vi "TestAll.vi"() -> ()   [LabVIEW 2016]
uses:
  Displacement/DisplacementErrorCodes.ctl
  Inclinometer/InclinometerErrorCodes.ctl
  Telemetry/TelemetryFields.ctl
  <vilib>/rvi/Emulation/niFpgaGetClockAttributes.vi
  <vilib>/rvi/Emulation/niFpgaSctlEmulationGetInTimedLoop.vi
  <vilib>/rvi/Emulation/niFpgaEmulationReportErrorSimple.vi
  <vilib>/rvi/Emulation/niFpgaProcessEmulError.vi
  <vilib>/rvi/Emulation/niFpgaEmulationIsFPGAContextNoSignature.vi
  <vilib>/rvi/errors/niFpgaSetErrorForExecOnDevCompSimple.vi
  <vilib>/rvi/eio/common/nirviEmuReportErrorAndStop.vi
  <vilib>/rvi/DataTransferAndStorage/Container/Common/niFpgaContainerGetUniqueNameForEmu.vi
  <vilib>/rvi/FIFO/Fifo_Resource/nirvififoEmulationSetSize.vi
  <vilib>/rvi/FIFO/Fifo_Resource/nirviFifoEmulationQueueMgr.vi
  <instcachedir>/0/nirviFifoEmulationQueueMgr_E5CAEC123FF24DC58D834DCA3CDAA9B5.lvgen/nirviFifoEmulationQueueMgr_E5CAEC123FF24DC58D834DCA3CDAA9B5_004.vi
  <vilib>/rvi/FIFO/Fifo_Resource/nirvififoEmulationDetermineInputValidOut.vi
  <vilib>/rvi/FIFO/Fifo_Resource/nirvififoEmulationCreateLock.vi
  <vilib>/rvi/FIFO/Fifo_Resource/nirvififoEmulationObtainLock.vi
  <vilib>/rvi/FIFO/Fifo_Resource/nirvififoEmulationReleaseLock.vi
  <vilib>/rvi/occurrence/nirviWaitOnOccurrenceBase.vi
  <vilib>/rvi/errors/nirviReportUnexpectedCaseInternalError.vi
  <vilib>/rvi/errors/nirviReportUnexpectedCaseInternalError (U32).vi
  <vilib>/Utility/error.llb/Clear Errors.vi
  <vilib>/rvi/Emulation/niFpgaCriticalErrorInLSC.vi
  <vilib>/rvi/Memory/Memory_Emulation/nirvimemoryFastEmulation.vi
  <vilib>/rvi/Memory/Memory_Emulation/nirvimemoryEmulation.vi
  <vilib>/rvi/DataTransferAndStorage/Container/Common/niFpgaContainerExecOnDevCompGetState.vi
  <vilib>/rvi/Memory/Memory_Emulation/niFpgaMemoryEmulationCacheClearOnFirstRun.vi
  <vilib>/rvi/Memory/Memory_Emulation/nirvimemoryEmulationManagerCache_MakeExclusive.vi
  <vilib>/rvi/Memory/Memory_Emulation/niFpgaMemoryEmulationValidateCache.vi
  <vilib>/rvi/Memory/Memory_Emulation/nirvimemoryEmulationManagerCache_InsertValue.vi
  <vilib>/rvi/Memory/Memory_Emulation/nirvimemoryEmulationManagerCache_ReleaseExclusive.vi
  <vilib>/rvi/Memory/Memory_Emulation/nirvimemoryEmulationManagerCache_GetValue.vi
  <vilib>/rvi/Memory/Memory_Emulation/nirvimemoryEmulationManagerCache_SetValue.vi
  <vilib>/rvi/Emulation/niFpgaSctlEmulationResourceMgr.vi
  <instcachedir>/0/nirviFifoEmulationQueueMgr_E5CAEC123FF24DC58D834DCA3CDAA9B5.lvgen/nirviFifoEmulationQueueMgr_E5CAEC123FF24DC58D834DCA3CDAA9B5_043.vi
  <instcachedir>/0/nirviFifoEmulationQueueMgr_E5CAEC123FF24DC58D834DCA3CDAA9B5.lvgen/nirviFifoEmulationQueueMgr_E5CAEC123FF24DC58D834DCA3CDAA9B5_040.vi
  <instcachedir>/0/nirviFifoEmulationQueueMgr_E5CAEC123FF24DC58D834DCA3CDAA9B5.lvgen/nirviFifoEmulationQueueMgr_E5CAEC123FF24DC58D834DCA3CDAA9B5_041.vi
  <instcachedir>/0/nirviFifoEmulationQueueMgr_E5CAEC123FF24DC58D834DCA3CDAA9B5.lvgen/nirviFifoEmulationQueueMgr_E5CAEC123FF24DC58D834DCA3CDAA9B5_042.vi
  <instcachedir>/0/nirviFifoEmulationQueueMgr_E5CAEC123FF24DC58D834DCA3CDAA9B5.lvgen/nirviFifoEmulationQueueMgr_E5CAEC123FF24DC58D834DCA3CDAA9B5_038.vi
  <vilib>/rvi/DataTransferAndStorage/Container/XNode/niFpgaContainer.xnode
  <vilib>/rvi/FIFO/Fifo_Resource/nirvififoEmulationWrite.vi
  <vilib>/rvi/FIFO/Fifo_Resource/nirvififoEmulationRead.vi
  <vilib>/rvi/Memory/Memory_Emulation/niFpgaMemoryEmulationRefIn.vi
panel:
  out "Step":i32
  out "Iteration":i32
  out "InclinometerErrorCodeTimestamp":u64
  out "InclinometerSampleTimestamp":u64
  out "InclinometerRxFrames":u64
  out "InclinometerTxFrames":u64
  out "InclinometerRxBytes":u64
  out "InclinometerTxBytes":u64
  out "InclinometerZenithAngle":sgl
  out "InclinometerRawAngle":u32
  out "InclinometerErrorCode":T1
  out "DisplacementErrorCode":T2
  out "DisplacementErrorTimestamp":u64
  out "DisplacementRotationZ":sgl
  out "DisplacementRotationY":sgl
  out "DisplacementRotationX":sgl
  out "DisplacementPositionZ":sgl
  out "DisplacementPositionY":sgl
  out "DisplacementPositionX":sgl
  out "DisplacementEng8":sgl
  out "DisplacementEng7":sgl
  out "DisplacementEng6":sgl
  out "DisplacementEng5":sgl
  out "DisplacementEng4":sgl
  out "DisplacementEng3":sgl
  out "DisplacementEng2":sgl
  out "DisplacementEng1":sgl
  out "DisplacementRaw8":i32
  out "DisplacementRaw7":i32
  out "DisplacementRaw6":i32
  out "DisplacementRaw5":i32
  out "DisplacementRaw4":i32
  out "DisplacementRaw3":i32
  out "DisplacementRaw2":i32
  out "DisplacementRaw1":i32
  out "DisplacementSampleTimestamp":u64
  out "DisplacementRxFrames":u64
  out "DisplacementTxFrames":u64
  out "DisplacementRxBytes":u64
  out "DisplacementTxBytes":u64
  out "AngularAccelerationZ":sgl format="%#.6f"
  out "AngularAccelerationY":sgl format="%#.6f"
  out "AngularAccelerationX":sgl format="%#.6f"
  out "AccelerometerEng8":sgl format="%#.6f"
  out "AccelerometerEng7":sgl format="%#.6f"
  out "AccelerometerEng6":sgl format="%#.6f"
  out "AccelerometerEng5":sgl format="%#.6f"
  out "AccelerometerEng4":sgl format="%#.6f"
  out "AccelerometerEng3":sgl format="%#.6f"
  out "AccelerometerEng2":sgl format="%#.6f"
  out "AccelerometerEng1":sgl format="%#.6f"
  out "AccelerometerTimestamp":u64
  out "AccelerometerRaw1":sgl format="%#.6f"
  out "AccelerometerRaw2":sgl format="%#.6f"
  out "AccelerometerRaw3":sgl format="%#.6f"
  out "AccelerometerRaw4":sgl format="%#.6f"
  out "AccelerometerRaw5":sgl format="%#.6f"
  out "AccelerometerRaw6":sgl format="%#.6f"
  out "AccelerometerRaw7":sgl format="%#.6f"
  out "AccelerometerRaw8":sgl format="%#.6f"
  out "AccelerometerSampleCount":u64
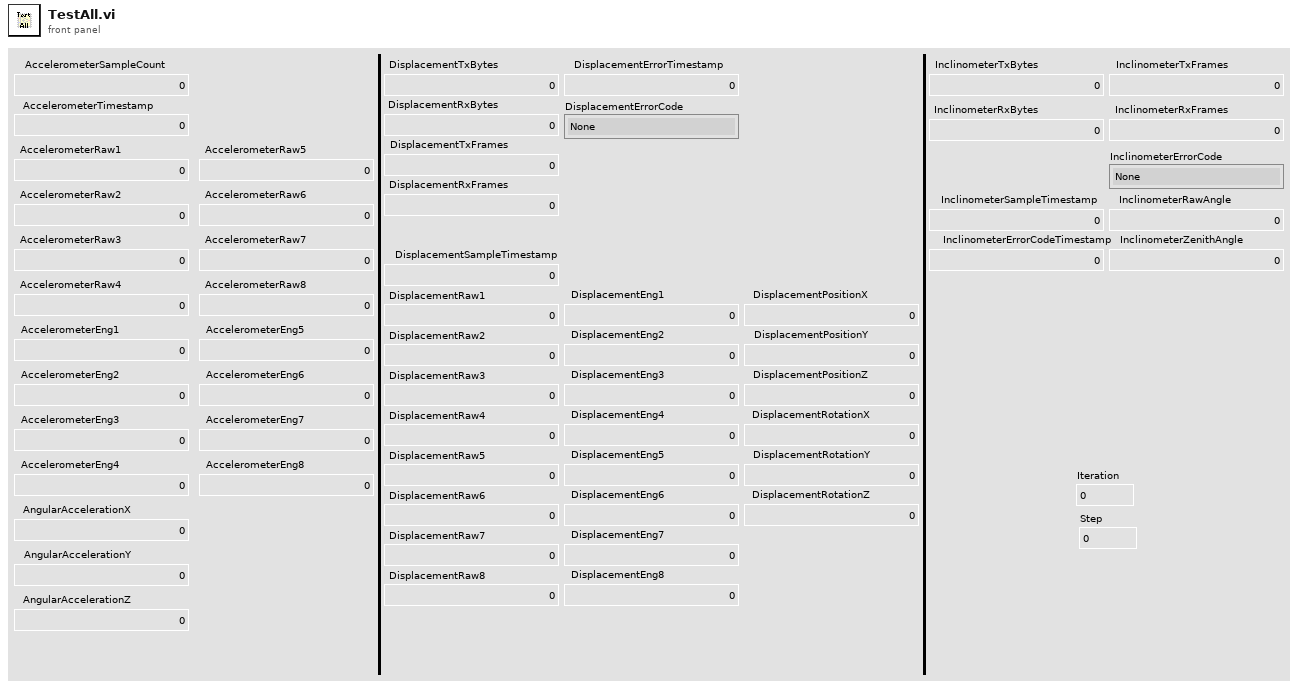
[diagram p1: front panel]
types:
  T1 = typedef "InclinometerErrorCodes.ctl" = enum8{"None", "ResponseAddressError", "ResponseFunctionCodeError", "ResponseByteCountError", "ResponseCRCError", "ResponseUnknownError", "ResponseTimeoutError", "SensorReportsIllegalFunction", "SensorReportsIllegalDataAddress"}
  T2 = typedef "DisplacementErrorCodes.ctl" = enum16{"None", "ResponseUnknownError", "ResponseInvalidError", "ResponseTimeoutError", "SensorIndicatesInvalidCommandError", "SensorIndicatesCommunicationTimeoutError", "SensorIndicatesDataLengthError", "SensorIndicatesNumberOfParametersError", "SensorIndicatesParameterError", "SensorIndicatesCommunicationError", "SensorIndicatesIDNumberError", "SensorIndicatesExpansionLineError", "SensorIndicatesWriteControlError"}
  T3 = cluster{"Timestamp":u64, "TxBytes":u64, "RxBytes":u64, "TxFrames":u64, "RxFrames":u64, "GyroX":u32, "GyroY":u32, "GyroZ":u32, "Status":u8, "SequenceNumber":u8, "Temperature":i16}
  T4 = cluster{"Timestamp":u64, "TxBytes":u64, "RxBytes":u64, "TxFrames":u64, "RxFrames":u64, "BIT0":u8, "BIT1":u8, "BIT2":u8, "BIT3":u8, "BIT4":u8, "BIT5":u8, "BIT6":u8, "BIT7":u8}
  T5 = cluster{"Timestamp":u64, "TxBytes":u64, "RxBytes":u64, "TxFrames":u64, "RxFrames":u64, "BIT0":u8, "BIT1":u8, "BIT2":u8, "BIT3":u8, "BIT4":u8, "BIT5":u8}
  T6 = cluster{"Timestamp":u64, "TxBytes":u64, "RxBytes":u64, "TxFrames":u64, "RxFrames":u64, "ErrorCode":enum8{"None", "ResponseHeaderError", "ResponseCRCError", "ResponseTimeoutError", "ResponseChecksumError"}}
  T7 = typedef "TelemetryFields.ctl" = enum16{"None", "InclinometerTxBytes", "InclinometerRxBytes", "InclinometerTxFrames", "InclinometerRxFrames", "InclinometerErrorTimestamp", "InclinometerErrorCode", "InclinometerSampleTimestamp", "InclinometerRawAngle", "InclinometerZenithAngle", "DisplacementTxBytes", "DisplacementRxBytes", "DisplacementTxFrames", "DisplacementRxFrames", "DisplacementErrorTimestamp", "DisplacementErrorCode", "DisplacementSampleTimestamp", "DisplacementRaw1", "DisplacementRaw2", "DisplacementRaw3", "DisplacementRaw4", "DisplacementRaw5", "DisplacementRaw6", "DisplacementRaw7", "DisplacementRaw8", "DisplacementEng1", "DisplacementEng2", "DisplacementEng3", "DisplacementEng4", "DisplacementEng5", "DisplacementEng6", "DisplacementEng7", "DisplacementEng8", "DisplacementPositionX", "DisplacementPositionY", "DisplacementPositionZ", "DisplacementRotationX", "DisplacementRotationY", "DisplacementRotationZ", "AccelerometerSampleCount", "AccelerometerSampleTimestamp", "AccelerometerRaw1", "AccelerometerRaw2", "AccelerometerRaw3", "AccelerometerRaw4", "AccelerometerRaw5", "AccelerometerRaw6", "AccelerometerRaw7", "AccelerometerRaw8", "AccelerometerEng1", "AccelerometerEng2", "AccelerometerEng3", "AccelerometerEng4", "AccelerometerEng5", "AccelerometerEng6", "AccelerometerEng7", "AccelerometerEng8", "AngularAccelerationX", "AngularAccelerationY", "AngularAccelerationZ", "GyroTxBytes", "GyroRxBytes", "GyroTxFrames", "GyroRxFrames", "GyroErrorTimestamp", "GyroErrorCode", "GyroSampleTimestamp", "AngularVelocityX", "AngularVelocityY", "AngularVelocityZ", "GyroStatus", "GyroSequenceNumber", "GyroTemperature", "GyroBITTimestamp", "GyroBIT0", "GyroBIT1", "GyroBIT2", "GyroBIT3", "GyroBIT4", "GyroBIT5", "GyroBIT6", "GyroBIT7"}
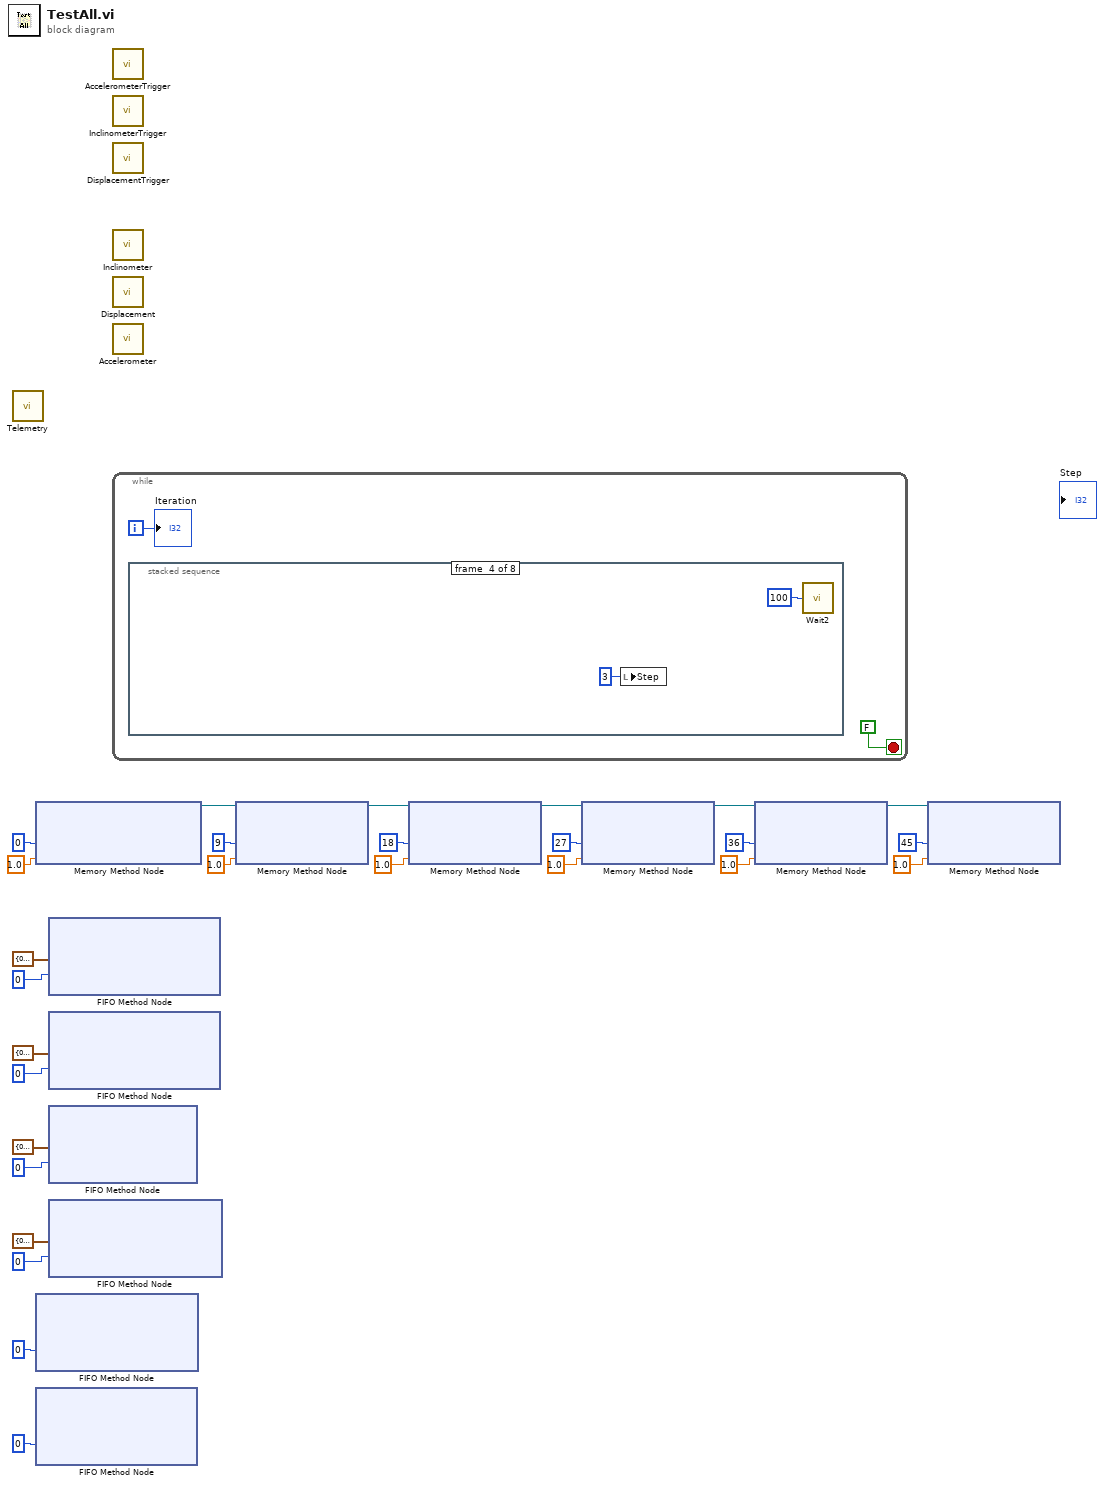
[diagram p0: block diagram]
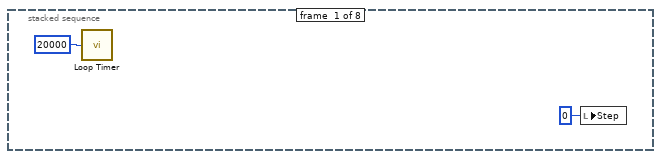
[diagram p2: hidden frame]
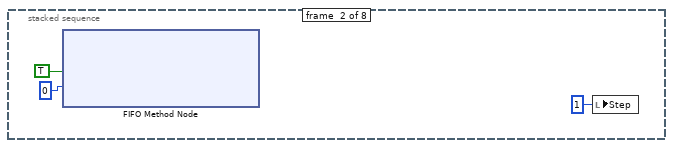
[diagram p3: hidden frame]
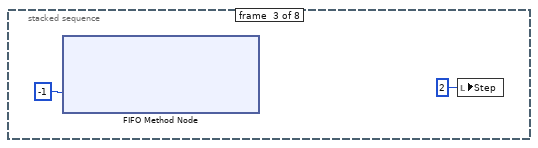
[diagram p4: hidden frame]
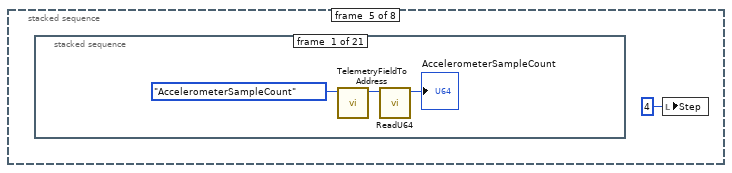
[diagram p5: hidden frame]
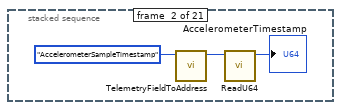
[diagram p6: hidden frame]
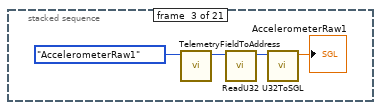
[diagram p7: hidden frame]
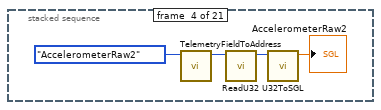
[diagram p8: hidden frame]
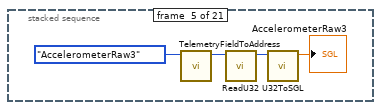
[diagram p9: hidden frame]
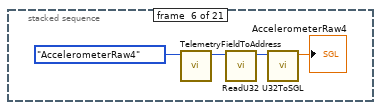
[diagram p10: hidden frame]
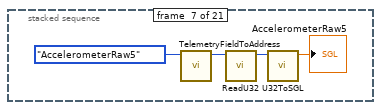
[diagram p11: hidden frame]
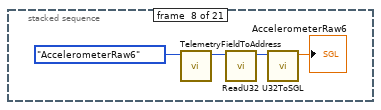
[diagram p12: hidden frame]
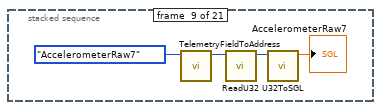
[diagram p13: hidden frame]
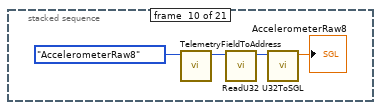
[diagram p14: hidden frame]
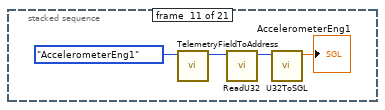
[diagram p15: hidden frame]
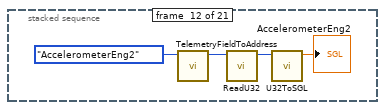
[diagram p16: hidden frame]
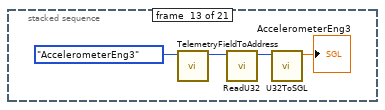
[diagram p17: hidden frame]
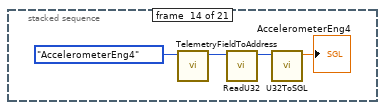
[diagram p18: hidden frame]
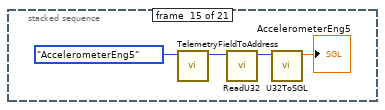
[diagram p19: hidden frame]
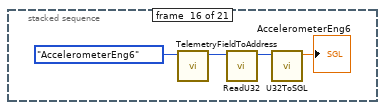
[diagram p20: hidden frame]
diagram:
  n1 = call "Telemetry.vi"() -> ()  [unwired: 12 in]
  n2 = xnode ("Memory Method Node")("Address"=u32 0, "Data"=sgl 1.0) -> ("Memory Out"=w21:refnum<k21>)  [unwired: 1 in]
  n3 = xnode ("FIFO Method Node")("Timeout"=0) -> ()  [unwired: 1 in, 3 out]
  n4 = xnode ("FIFO Method Node")("Timeout"=0) -> ()  [unwired: 1 in, 3 out]
  n5 = xnode ("FIFO Method Node")("Element"=T5 {"Timestamp"=0, "TxBytes"=0, "RxBytes"=0, "TxFrames"=0, "RxFrames"=0, "BIT0"=0, "BIT1"=0, "BIT2"=0, "BIT3"=0, "BIT4"=0, "BIT5"=0}, "Timeout"=0) -> ()  [unwired: 1 in, 2 out]
  n6 = xnode ("FIFO Method Node")("Element"=T4 {"Timestamp"=0, "TxBytes"=0, "RxBytes"=0, "TxFrames"=0, "RxFrames"=0, "BIT0"=0, "BIT1"=0, "BIT2"=0, "BIT3"=0, "BIT4"=0, "BIT5"=0, "BIT6"=0, "BIT7"=0}, "Timeout"=0) -> ()  [unwired: 1 in, 2 out]
  n7 = xnode ("FIFO Method Node")("Element"=T3 {"Timestamp"=0, "TxBytes"=0, "RxBytes"=0, "TxFrames"=0, "RxFrames"=0, "GyroX"=0, "GyroY"=0, "GyroZ"=0, "Status"=0, "SequenceNumber"=0, "Temperature"=0}, "Timeout"=0) -> ()  [unwired: 1 in, 2 out]
  n8 = xnode ("FIFO Method Node")("Element"=T6 {"Timestamp"=0, "TxBytes"=0, "RxBytes"=0, "TxFrames"=0, "RxFrames"=0, "ErrorCode"=enum."None"}, "Timeout"=0) -> ()  [unwired: 1 in, 2 out]
  n9 = call "AccelerometerTrigger.vi"() -> ()  [unwired: 12 in]
  n10 = call "InclinometerTrigger.vi"() -> ()  [unwired: 12 in]
  n11 = call "DisplacementTrigger.vi"() -> ()  [unwired: 12 in]
  n12 = call "Inclinometer.vi"() -> ()  [unwired: 12 in]
  n13 = call "Displacement.vi"() -> ()  [unwired: 12 in]
  n14 = call "Accelerometer.vi"() -> ()  [unwired: 12 in]
  n15 = while {
    i -> [w28]
    stop <- FALSE stop-if-true
    n16 = stacked-sequence {
      frame #0 {
        n17 = call "Loop Timer"("Count(uSec)"=u32 20000) -> ()  [unwired: 1 out]
        n18 = local write "Step"(0 ("Step")) -> ()
      }
      frame #1 {
        n19 = xnode ("FIFO Method Node")("Element"=TRUE, "Timeout"=0) -> ()  [unwired: 1 in, 2 out]
        n20 = local write "Step"(1 ("Step")) -> ()
      }
      frame #2 {
        n21 = xnode ("FIFO Method Node")("Timeout"=-1) -> ()  [unwired: 1 in, 3 out]
        n22 = local write "Step"(2 ("Step")) -> ()
      }
      frame #3 {
        n23 = local write "Step"(3 ("Step")) -> ()
        n24 = call "Wait2"("Count(uSec)"=u32 100) -> ()  [unwired: 1 out]
      }
      frame #4 {
        n25 = stacked-sequence {
          frame #0 {
            n26 = call "TelemetryFieldToAddress.vi"("TelemetryFields"=TelemetryFields."AccelerometerSampleCount") -> ("Address"=w41:u32)  [unwired: 10 in]
            n27 = call "ReadU64.vi"("Address"=w41) -> ("Data"=→"AccelerometerSampleCount":u64)  [unwired: 10 in]
          }
          frame #1 {
            n28 = call "TelemetryFieldToAddress.vi"("TelemetryFields"=TelemetryFields."AccelerometerSampleTimestamp") -> ("Address"=w45:u32)  [unwired: 10 in]
            n29 = call "ReadU64.vi"("Address"=w45) -> ("Data"=→"AccelerometerTimestamp":u64)  [unwired: 10 in]
          }
          frame #2 {
            n30 = call "TelemetryFieldToAddress.vi"("TelemetryFields"=TelemetryFields."AccelerometerRaw1") -> ("Address"=w49:u32)  [unwired: 10 in]
            n31 = call "ReadU32.vi"("Address"=w49) -> ("Data"=w48:u32)  [unwired: 10 in]
            n32 = call "U32ToSGL.vi"("U32"=w48) -> ("SGL"=→"AccelerometerRaw1":sgl)  [unwired: 10 in]
          }
          frame #3 {
            n33 = call "TelemetryFieldToAddress.vi"("TelemetryFields"=TelemetryFields."AccelerometerRaw2") -> ("Address"=w53:u32)  [unwired: 10 in]
            n34 = call "ReadU32.vi"("Address"=w53) -> ("Data"=w52:u32)  [unwired: 10 in]
            n35 = call "U32ToSGL.vi"("U32"=w52) -> ("SGL"=→"AccelerometerRaw2":sgl)  [unwired: 10 in]
          }
          frame #4 {
            n36 = call "TelemetryFieldToAddress.vi"("TelemetryFields"=TelemetryFields."AccelerometerRaw3") -> ("Address"=w57:u32)  [unwired: 10 in]
            n37 = call "ReadU32.vi"("Address"=w57) -> ("Data"=w56:u32)  [unwired: 10 in]
            n38 = call "U32ToSGL.vi"("U32"=w56) -> ("SGL"=→"AccelerometerRaw3":sgl)  [unwired: 10 in]
          }
          frame #5 {
            n39 = call "TelemetryFieldToAddress.vi"("TelemetryFields"=TelemetryFields."AccelerometerRaw4") -> ("Address"=w61:u32)  [unwired: 10 in]
            n40 = call "ReadU32.vi"("Address"=w61) -> ("Data"=w60:u32)  [unwired: 10 in]
            n41 = call "U32ToSGL.vi"("U32"=w60) -> ("SGL"=→"AccelerometerRaw4":sgl)  [unwired: 10 in]
          }
          frame #6 {
            n42 = call "TelemetryFieldToAddress.vi"("TelemetryFields"=TelemetryFields."AccelerometerRaw5") -> ("Address"=w65:u32)  [unwired: 10 in]
            n43 = call "ReadU32.vi"("Address"=w65) -> ("Data"=w64:u32)  [unwired: 10 in]
            n44 = call "U32ToSGL.vi"("U32"=w64) -> ("SGL"=→"AccelerometerRaw5":sgl)  [unwired: 10 in]
          }
          frame #7 {
            n45 = call "TelemetryFieldToAddress.vi"("TelemetryFields"=TelemetryFields."AccelerometerRaw6") -> ("Address"=w69:u32)  [unwired: 10 in]
            n46 = call "ReadU32.vi"("Address"=w69) -> ("Data"=w68:u32)  [unwired: 10 in]
            n47 = call "U32ToSGL.vi"("U32"=w68) -> ("SGL"=→"AccelerometerRaw6":sgl)  [unwired: 10 in]
          }
          frame #8 {
            n48 = call "TelemetryFieldToAddress.vi"("TelemetryFields"=TelemetryFields."AccelerometerRaw7") -> ("Address"=w73:u32)  [unwired: 10 in]
            n49 = call "ReadU32.vi"("Address"=w73) -> ("Data"=w72:u32)  [unwired: 10 in]
            n50 = call "U32ToSGL.vi"("U32"=w72) -> ("SGL"=→"AccelerometerRaw7":sgl)  [unwired: 10 in]
          }
          frame #9 {
            n51 = call "TelemetryFieldToAddress.vi"("TelemetryFields"=TelemetryFields."AccelerometerRaw8") -> ("Address"=w77:u32)  [unwired: 10 in]
            n52 = call "ReadU32.vi"("Address"=w77) -> ("Data"=w76:u32)  [unwired: 10 in]
            n53 = call "U32ToSGL.vi"("U32"=w76) -> ("SGL"=→"AccelerometerRaw8":sgl)  [unwired: 10 in]
          }
          frame #10 {
            n54 = call "TelemetryFieldToAddress.vi"("TelemetryFields"=TelemetryFields."AccelerometerEng1") -> ("Address"=w81:u32)  [unwired: 10 in]
            n55 = call "ReadU32.vi"("Address"=w81) -> ("Data"=w80:u32)  [unwired: 10 in]
            n56 = call "U32ToSGL.vi"("U32"=w80) -> ("SGL"=→"AccelerometerEng1":sgl)  [unwired: 10 in]
          }
          frame #11 {
            n57 = call "TelemetryFieldToAddress.vi"("TelemetryFields"=TelemetryFields."AccelerometerEng2") -> ("Address"=w85:u32)  [unwired: 10 in]
            n58 = call "ReadU32.vi"("Address"=w85) -> ("Data"=w84:u32)  [unwired: 10 in]
            n59 = call "U32ToSGL.vi"("U32"=w84) -> ("SGL"=→"AccelerometerEng2":sgl)  [unwired: 10 in]
          }
          frame #12 {
            n60 = call "TelemetryFieldToAddress.vi"("TelemetryFields"=TelemetryFields."AccelerometerEng3") -> ("Address"=w89:u32)  [unwired: 10 in]
            n61 = call "ReadU32.vi"("Address"=w89) -> ("Data"=w88:u32)  [unwired: 10 in]
            n62 = call "U32ToSGL.vi"("U32"=w88) -> ("SGL"=→"AccelerometerEng3":sgl)  [unwired: 10 in]
          }
          frame #13 {
            n63 = call "TelemetryFieldToAddress.vi"("TelemetryFields"=TelemetryFields."AccelerometerEng4") -> ("Address"=w93:u32)  [unwired: 10 in]
            n64 = call "ReadU32.vi"("Address"=w93) -> ("Data"=w92:u32)  [unwired: 10 in]
            n65 = call "U32ToSGL.vi"("U32"=w92) -> ("SGL"=→"AccelerometerEng4":sgl)  [unwired: 10 in]
          }
          frame #14 {
            n66 = call "TelemetryFieldToAddress.vi"("TelemetryFields"=TelemetryFields."AccelerometerEng5") -> ("Address"=w97:u32)  [unwired: 10 in]
            n67 = call "ReadU32.vi"("Address"=w97) -> ("Data"=w96:u32)  [unwired: 10 in]
            n68 = call "U32ToSGL.vi"("U32"=w96) -> ("SGL"=→"AccelerometerEng5":sgl)  [unwired: 10 in]
          }
          frame #15 {
            n69 = call "TelemetryFieldToAddress.vi"("TelemetryFields"=TelemetryFields."AccelerometerEng6") -> ("Address"=w101:u32)  [unwired: 10 in]
            n70 = call "ReadU32.vi"("Address"=w101) -> ("Data"=w100:u32)  [unwired: 10 in]
            n71 = call "U32ToSGL.vi"("U32"=w100) -> ("SGL"=→"AccelerometerEng6":sgl)  [unwired: 10 in]
          }
          frame #16 {
            n72 = call "TelemetryFieldToAddress.vi"("TelemetryFields"=TelemetryFields."AccelerometerEng7") -> ("Address"=w105:u32)  [unwired: 10 in]
            n73 = call "ReadU32.vi"("Address"=w105) -> ("Data"=w104:u32)  [unwired: 10 in]
            n74 = call "U32ToSGL.vi"("U32"=w104) -> ("SGL"=→"AccelerometerEng7":sgl)  [unwired: 10 in]
          }
          frame #17 {
            n75 = call "TelemetryFieldToAddress.vi"("TelemetryFields"=TelemetryFields."AccelerometerEng8") -> ("Address"=w109:u32)  [unwired: 10 in]
            n76 = call "ReadU32.vi"("Address"=w109) -> ("Data"=w108:u32)  [unwired: 10 in]
            n77 = call "U32ToSGL.vi"("U32"=w108) -> ("SGL"=→"AccelerometerEng8":sgl)  [unwired: 10 in]
          }
          frame #18 {
            n78 = call "TelemetryFieldToAddress.vi"("TelemetryFields"=TelemetryFields."AngularAccelerationX") -> ("Address"=w113:u32)  [unwired: 10 in]
            n79 = call "ReadU32.vi"("Address"=w113) -> ("Data"=w112:u32)  [unwired: 10 in]
            n80 = call "U32ToSGL.vi"("U32"=w112) -> ("SGL"=→"AngularAccelerationX":sgl)  [unwired: 10 in]
          }
          frame #19 {
            n81 = call "TelemetryFieldToAddress.vi"("TelemetryFields"=TelemetryFields."AngularAccelerationY") -> ("Address"=w117:u32)  [unwired: 10 in]
            n82 = call "ReadU32.vi"("Address"=w117) -> ("Data"=w116:u32)  [unwired: 10 in]
            n83 = call "U32ToSGL.vi"("U32"=w116) -> ("SGL"=→"AngularAccelerationY":sgl)  [unwired: 10 in]
          }
          frame #20 {
            n84 = call "TelemetryFieldToAddress.vi"("TelemetryFields"=TelemetryFields."AngularAccelerationZ") -> ("Address"=w121:u32)  [unwired: 10 in]
            n85 = call "ReadU32.vi"("Address"=w121) -> ("Data"=w120:u32)  [unwired: 10 in]
            n86 = call "U32ToSGL.vi"("U32"=w120) -> ("SGL"=→"AngularAccelerationZ":sgl)  [unwired: 10 in]
          }
        }
        n87 = local write "Step"(4 ("Step")) -> ()
      }
      frame #5 {
        n88 = stacked-sequence {
          frame #0 {
            n89 = call "TelemetryFieldToAddress.vi"("TelemetryFields"=TelemetryFields."DisplacementTxBytes") -> ("Address"=w123:u32)  [unwired: 10 in]
            n90 = call "ReadU64.vi"("Address"=w123) -> ("Data"=→"DisplacementTxBytes":u64)  [unwired: 10 in]
          }
          frame #1 {
            n91 = call "TelemetryFieldToAddress.vi"("TelemetryFields"=TelemetryFields."DisplacementRxBytes") -> ("Address"=w128:u32)  [unwired: 10 in]
            n92 = call "ReadU64.vi"("Address"=w128) -> ("Data"=→"DisplacementRxBytes":u64)  [unwired: 10 in]
          }
          frame #2 {
            n93 = call "TelemetryFieldToAddress.vi"("TelemetryFields"=TelemetryFields."DisplacementTxFrames") -> ("Address"=w129:u32)  [unwired: 10 in]
            n94 = call "ReadU64.vi"("Address"=w129) -> ("Data"=→"DisplacementTxFrames":u64)  [unwired: 10 in]
          }
          frame #3 {
            n95 = call "TelemetryFieldToAddress.vi"("TelemetryFields"=TelemetryFields."DisplacementRxFrames") -> ("Address"=w134:u32)  [unwired: 10 in]
            n96 = call "ReadU64.vi"("Address"=w134) -> ("Data"=→"DisplacementRxFrames":u64)  [unwired: 10 in]
          }
          frame #4 {
            n97 = call "TelemetryFieldToAddress.vi"("TelemetryFields"=TelemetryFields."DisplacementSampleTimestamp") -> ("Address"=w137:u32)  [unwired: 10 in]
            n98 = call "ReadU64.vi"("Address"=w137) -> ("Data"=→"DisplacementSampleTimestamp":u64)  [unwired: 10 in]
          }
          frame #5 {
            n99 = call "TelemetryFieldToAddress.vi"("TelemetryFields"=TelemetryFields."DisplacementRaw1") -> ("Address"=w138:u32)  [unwired: 10 in]
            n100 = call "ReadI32.vi"("Address"=w138) -> ("Data"=→"DisplacementRaw1":i32)  [unwired: 10 in]
          }
          frame #6 {
            n101 = call "TelemetryFieldToAddress.vi"("TelemetryFields"=TelemetryFields."DisplacementRaw2") -> ("Address"=w143:u32)  [unwired: 10 in]
            n102 = call "ReadI32.vi"("Address"=w143) -> ("Data"=→"DisplacementRaw2":i32)  [unwired: 10 in]
          }
          frame #7 {
            n103 = call "TelemetryFieldToAddress.vi"("TelemetryFields"=TelemetryFields."DisplacementRaw3") -> ("Address"=w144:u32)  [unwired: 10 in]
            n104 = call "ReadI32.vi"("Address"=w144) -> ("Data"=→"DisplacementRaw3":i32)  [unwired: 10 in]
          }
          frame #8 {
            n105 = call "TelemetryFieldToAddress.vi"("TelemetryFields"=TelemetryFields."DisplacementRaw4") -> ("Address"=w149:u32)  [unwired: 10 in]
            n106 = call "ReadI32.vi"("Address"=w149) -> ("Data"=→"DisplacementRaw4":i32)  [unwired: 10 in]
          }
          frame #9 {
            n107 = call "TelemetryFieldToAddress.vi"("TelemetryFields"=TelemetryFields."DisplacementRaw5") -> ("Address"=w150:u32)  [unwired: 10 in]
            n108 = call "ReadI32.vi"("Address"=w150) -> ("Data"=→"DisplacementRaw5":i32)  [unwired: 10 in]
          }
          frame #10 {
            n109 = call "TelemetryFieldToAddress.vi"("TelemetryFields"=TelemetryFields."DisplacementRaw6") -> ("Address"=w155:u32)  [unwired: 10 in]
            n110 = call "ReadI32.vi"("Address"=w155) -> ("Data"=→"DisplacementRaw6":i32)  [unwired: 10 in]
          }
          frame #11 {
            n111 = call "TelemetryFieldToAddress.vi"("TelemetryFields"=TelemetryFields."DisplacementRaw7") -> ("Address"=w156:u32)  [unwired: 10 in]
            n112 = call "ReadI32.vi"("Address"=w156) -> ("Data"=→"DisplacementRaw7":i32)  [unwired: 10 in]
          }
          frame #12 {
            n113 = call "TelemetryFieldToAddress.vi"("TelemetryFields"=TelemetryFields."DisplacementRaw8") -> ("Address"=w161:u32)  [unwired: 10 in]
            n114 = call "ReadI32.vi"("Address"=w161) -> ("Data"=→"DisplacementRaw8":i32)  [unwired: 10 in]
          }
          frame #13 {
            n115 = call "TelemetryFieldToAddress.vi"("TelemetryFields"=TelemetryFields."DisplacementEng1") -> ("Address"=w164:u32)  [unwired: 10 in]
            n116 = call "ReadSGL.vi"("Address"=w164) -> ("Data"=→"DisplacementEng1":sgl)  [unwired: 10 in]
          }
          frame #14 {
            n117 = call "TelemetryFieldToAddress.vi"("TelemetryFields"=TelemetryFields."DisplacementEng2") -> ("Address"=w165:u32)  [unwired: 10 in]
            n118 = call "ReadSGL.vi"("Address"=w165) -> ("Data"=→"DisplacementEng2":sgl)  [unwired: 10 in]
          }
          frame #15 {
            n119 = call "TelemetryFieldToAddress.vi"("TelemetryFields"=TelemetryFields."DisplacementEng3") -> ("Address"=w170:u32)  [unwired: 10 in]
            n120 = call "ReadSGL.vi"("Address"=w170) -> ("Data"=→"DisplacementEng3":sgl)  [unwired: 10 in]
          }
          frame #16 {
            n121 = call "TelemetryFieldToAddress.vi"("TelemetryFields"=TelemetryFields."DisplacementEng4") -> ("Address"=w171:u32)  [unwired: 10 in]
            n122 = call "ReadSGL.vi"("Address"=w171) -> ("Data"=→"DisplacementEng4":sgl)  [unwired: 10 in]
          }
          frame #17 {
            n123 = call "TelemetryFieldToAddress.vi"("TelemetryFields"=TelemetryFields."DisplacementEng5") -> ("Address"=w176:u32)  [unwired: 10 in]
            n124 = call "ReadSGL.vi"("Address"=w176) -> ("Data"=→"DisplacementEng5":sgl)  [unwired: 10 in]
          }
          frame #18 {
            n125 = call "TelemetryFieldToAddress.vi"("TelemetryFields"=TelemetryFields."DisplacementEng6") -> ("Address"=w177:u32)  [unwired: 10 in]
            n126 = call "ReadSGL.vi"("Address"=w177) -> ("Data"=→"DisplacementEng6":sgl)  [unwired: 10 in]
          }
          frame #19 {
            n127 = call "TelemetryFieldToAddress.vi"("TelemetryFields"=TelemetryFields."DisplacementEng7") -> ("Address"=w182:u32)  [unwired: 10 in]
            n128 = call "ReadSGL.vi"("Address"=w182) -> ("Data"=→"DisplacementEng7":sgl)  [unwired: 10 in]
          }
          frame #20 {
            n129 = call "TelemetryFieldToAddress.vi"("TelemetryFields"=TelemetryFields."DisplacementEng8") -> ("Address"=w185:u32)  [unwired: 10 in]
            n130 = call "ReadSGL.vi"("Address"=w185) -> ("Data"=→"DisplacementEng8":sgl)  [unwired: 10 in]
          }
          frame #21 {
            n131 = call "TelemetryFieldToAddress.vi"("TelemetryFields"=TelemetryFields."DisplacementPositionX") -> ("Address"=w186:u32)  [unwired: 10 in]
            n132 = call "ReadSGL.vi"("Address"=w186) -> ("Data"=→"DisplacementPositionX":sgl)  [unwired: 10 in]
          }
          frame #22 {
            n133 = call "TelemetryFieldToAddress.vi"("TelemetryFields"=TelemetryFields."DisplacementPositionY") -> ("Address"=w191:u32)  [unwired: 10 in]
            n134 = call "ReadSGL.vi"("Address"=w191) -> ("Data"=→"DisplacementPositionY":sgl)  [unwired: 10 in]
          }
          frame #23 {
            n135 = call "TelemetryFieldToAddress.vi"("TelemetryFields"=TelemetryFields."DisplacementPositionZ") -> ("Address"=w192:u32)  [unwired: 10 in]
            n136 = call "ReadSGL.vi"("Address"=w192) -> ("Data"=→"DisplacementPositionZ":sgl)  [unwired: 10 in]
          }
          frame #24 {
            n137 = call "TelemetryFieldToAddress.vi"("TelemetryFields"=TelemetryFields."DisplacementRotationX") -> ("Address"=w197:u32)  [unwired: 10 in]
            n138 = call "ReadSGL.vi"("Address"=w197) -> ("Data"=→"DisplacementRotationX":sgl)  [unwired: 10 in]
          }
          frame #25 {
            n139 = call "TelemetryFieldToAddress.vi"("TelemetryFields"=TelemetryFields."DisplacementRotationY") -> ("Address"=w198:u32)  [unwired: 10 in]
            n140 = call "ReadSGL.vi"("Address"=w198) -> ("Data"=→"DisplacementRotationY":sgl)  [unwired: 10 in]
          }
          frame #26 {
            n141 = call "TelemetryFieldToAddress.vi"("TelemetryFields"=TelemetryFields."DisplacementRotationZ") -> ("Address"=w203:u32)  [unwired: 10 in]
            n142 = call "ReadSGL.vi"("Address"=w203) -> ("Data"=→"DisplacementRotationZ":sgl)  [unwired: 10 in]
          }
          frame #27 {
            n143 = call "TelemetryFieldToAddress.vi"("TelemetryFields"=TelemetryFields."DisplacementErrorTimestamp") -> ("Address"=w204:u32)  [unwired: 10 in]
            n144 = call "ReadU64.vi"("Address"=w204) -> ("Data"=→"DisplacementErrorTimestamp":u64)  [unwired: 10 in]
          }
          frame #28 {
            n145 = call "TelemetryFieldToAddress.vi"("TelemetryFields"=TelemetryFields."DisplacementErrorCode") -> ("Address"=w208:u32)  [unwired: 10 in]
            n146 = call "ReadU8.vi"("Address"=w208) -> ("Data"=→"DisplacementErrorCode":u8)  [unwired: 10 in]
          }
        }
        n147 = local write "Step"(5 ("Step")) -> ()
      }
      frame #6 {
        n148 = stacked-sequence {
          frame #0 {
            n149 = call "TelemetryFieldToAddress.vi"("TelemetryFields"=TelemetryFields."InclinometerErrorCode") -> ("Address"=w213:u32)  [unwired: 10 in]
            n150 = call "ReadU8.vi"("Address"=w213) -> ("Data"=→"InclinometerErrorCode":u8)  [unwired: 10 in]
          }
          frame #1 {
            n151 = call "TelemetryFieldToAddress.vi"("TelemetryFields"=TelemetryFields."InclinometerRawAngle") -> ("Address"=w215:u32)  [unwired: 10 in]
            n152 = call "ReadU32.vi"("Address"=w215) -> ("Data"=→"InclinometerRawAngle":u32)  [unwired: 10 in]
          }
          frame #2 {
            n153 = call "TelemetryFieldToAddress.vi"("TelemetryFields"=TelemetryFields."InclinometerZenithAngle") -> ("Address"=w218:u32)  [unwired: 10 in]
            n154 = call "ReadSGL.vi"("Address"=w218) -> ("Data"=→"InclinometerZenithAngle":sgl)  [unwired: 10 in]
          }
          frame #3 {
            n155 = call "TelemetryFieldToAddress.vi"("TelemetryFields"=TelemetryFields."InclinometerTxBytes") -> ("Address"=w221:u32)  [unwired: 10 in]
            n156 = call "ReadU64.vi"("Address"=w221) -> ("Data"=→"InclinometerTxBytes":u64)  [unwired: 10 in]
          }
          frame #4 {
            n157 = call "TelemetryFieldToAddress.vi"("TelemetryFields"=TelemetryFields."InclinometerRxBytes") -> ("Address"=w224:u32)  [unwired: 10 in]
            n158 = call "ReadU64.vi"("Address"=w224) -> ("Data"=→"InclinometerRxBytes":u64)  [unwired: 10 in]
          }
          frame #5 {
            n159 = call "TelemetryFieldToAddress.vi"("TelemetryFields"=TelemetryFields."InclinometerTxFrames") -> ("Address"=w227:u32)  [unwired: 10 in]
            n160 = call "ReadU64.vi"("Address"=w227) -> ("Data"=→"InclinometerTxFrames":u64)  [unwired: 10 in]
          }
          frame #6 {
            n161 = call "TelemetryFieldToAddress.vi"("TelemetryFields"=TelemetryFields."InclinometerRxFrames") -> ("Address"=w230:u32)  [unwired: 10 in]
            n162 = call "ReadU64.vi"("Address"=w230) -> ("Data"=→"InclinometerRxFrames":u64)  [unwired: 10 in]
          }
          frame #7 {
            n163 = call "TelemetryFieldToAddress.vi"("TelemetryFields"=TelemetryFields."InclinometerSampleTimestamp") -> ("Address"=w233:u32)  [unwired: 10 in]
            n164 = call "ReadU64.vi"("Address"=w233) -> ("Data"=→"InclinometerSampleTimestamp":u64)  [unwired: 10 in]
          }
          frame #8 {
            n165 = call "TelemetryFieldToAddress.vi"("TelemetryFields"=TelemetryFields."InclinometerErrorTimestamp") -> ("Address"=w236:u32)  [unwired: 10 in]
            n166 = call "ReadU64.vi"("Address"=w236) -> ("Data"=→"InclinometerErrorCodeTimestamp":u64)  [unwired: 10 in]
          }
        }
        n167 = local write "Step"(6 ("Step")) -> ()
      }
      frame #7 {
        n168 = xnode ("FIFO Method Node")("Element"=TRUE, "Timeout"=0) -> ()  [unwired: 1 in, 2 out]
        n169 = local write "Step"(7 ("Step")) -> ()
      }
    }
    "Iteration" <- w28
  }
  n170 = xnode ("Memory Method Node")("Address"=u32 9, "Data"=sgl 1.0, "Memory In"=w21) -> ("Memory Out"=w20:refnum<k21>)
  n171 = xnode ("Memory Method Node")("Address"=u32 18, "Data"=sgl 1.0, "Memory In"=w20) -> ("Memory Out"=w13:refnum<k21>)
  n172 = xnode ("Memory Method Node")("Address"=u32 27, "Data"=sgl 1.0, "Memory In"=w13) -> ("Memory Out"=w12:refnum<k21>)
  n173 = xnode ("Memory Method Node")("Address"=u32 36, "Data"=sgl 1.0, "Memory In"=w12) -> ("Memory Out"=w11:refnum<k21>)
  n174 = xnode ("Memory Method Node")("Address"=u32 45, "Data"=sgl 1.0, "Memory In"=w11) -> ()  [unwired: 1 out]
